vi "Waveform Running Average.vi"(8 "Current Data Index":u64, 10 "Additional Data":waveform(dbl), 11 "Running Average In":waveform(dbl)) -> (3 "Running Average Out":waveform(dbl))   [LabVIEW 2009]
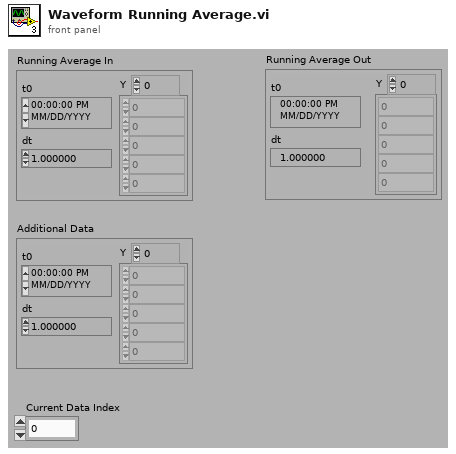
[diagram p1: front panel]
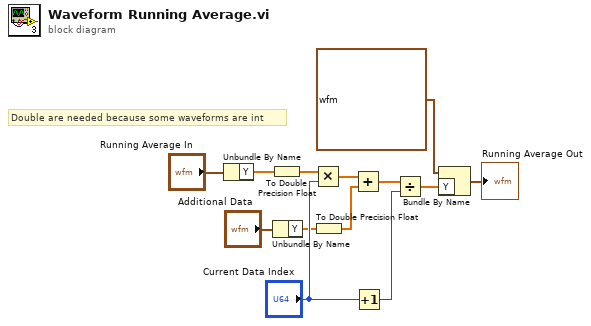
[diagram p0: block diagram]
diagram:
  # "Double are needed because some waveforms are int"
  n1 = Unbundle By Name("Running Average In") -> ("Y"=w4:dbl[])
  n2 = To Double Precision Float(number=w4) -> (double precision float=w3:dbl[])
  n3 = Unbundle By Name("Additional Data") -> ("Y"=w2:dbl[])
  n4 = Multiply(x=w3, y="Current Data Index") -> (x*y=w7:dbl[])
  n5 = To Double Precision Float(number=w2) -> (double precision float=w1:dbl[])
  n6 = Add(x=w7, y=w1) -> (x+y=w10:dbl[])
  n7 = Increment(x="Current Data Index") -> (x+1=w9:u64)
  n8 = Divide(x=w10, y=w9) -> (x/y=w6:dbl[])
  n9 = Bundle By Name(cluster=waveform(dbl) {"t0"=timestamp(0 s since 1904-01-01), "dt"=1.0, "Y"=[]} ("waveform"), "Y"=w6) -> (→"Running Average Out":waveform(dbl))
